vi "MIDAS_ODB_Find.vi"(8 "Array":T1[](array[typedef]), 11 "input cluster":T1) -> (2 "Found Entry":bool, 3 "MIDAS_ODB_Entry":T1)   [LabVIEW 2018, in "feGEM DataPacker.lvlib"]
uses:
  MIDAS_ODB_Entry.ctl
  feGEM DataPacker.lvlib
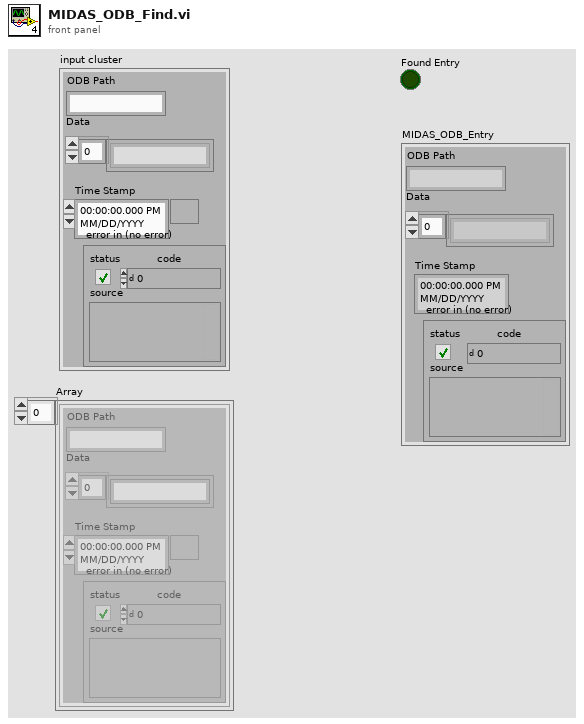
[diagram p1: front panel]
types:
  T1 = typedef "feGEM DataPacker.lvlib/MIDAS_ODB_Entry.ctl" = cluster{"ODB Path":string, "Data":string[], "Time Stamp":timestamp, "error in (no error)":errorcluster}
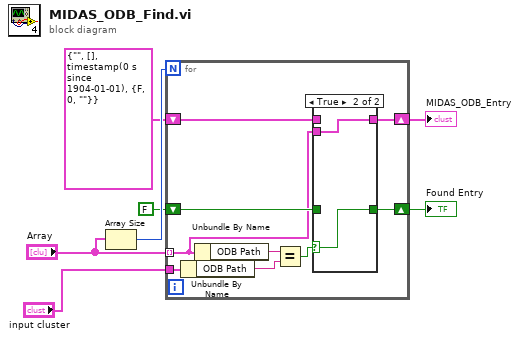
[diagram p0: block diagram]
diagram:
  n1 = Array Size(array="Array") -> (size(s)=w7:i32)
  n2 = for {
    N: w7 -> [_]
    tunnel: "Array" -> [w10] mode=indexing
    shift-right: [w14] -> w2
    shift-left: FALSE -> [w13]
    shift-right: [w11] -> w3
    shift-left: T1 {"ODB Path"="", "Data"=[], "Time Stamp"=timestamp(0 s since 1904-01-01), "error in (no error)"={"status"=FALSE, "code"=0, "source"=""}} ("input cluster") -> [w12]
    tunnel: "input cluster" -> [w8]
    n3 = Unbundle By Name(w8) -> ("ODB Path"=w9:string)
    n4 = Unbundle By Name(w10) -> ("ODB Path"=w16:string)
    n5 = Equal?(x=w16, y=w9) -> (x = y?=w15:bool)
    n6 = case shown="True" w15 {
      selector: w15 -> [_ w20]
      tunnel: [w18 w20] -> w14
      tunnel: w13 -> [w18 _]
      tunnel: w12 -> [w17 _]
      tunnel: [w17 w19] -> w11
      tunnel: w10 -> [_ w19]
      frame False {
      }
      frame True {
      }
    }
  }
  "Found Entry" <- w2
  "MIDAS_ODB_Entry" <- w3
